vi "InitEqui.vi"(8 "errin":errorcluster, 10 "VISA HITECH":string, 11 "VISA Auto":string) -> (0 "errout":errorcluster, 2 "VisaHitech":refnum<visa-resource-name>, 3 "VISA Refnum out":refnum<visa-resource-name>)   [LabVIEW 2020]
uses:
  <vilib>/Instr/_visa.llb/VISA Configure Serial Port (Instr).vi
  <instrlib>/IT6000C/IT6000C.lvlib
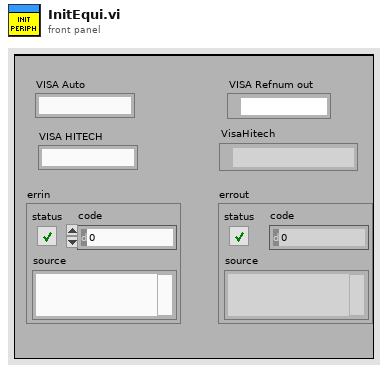
[diagram p1: front panel]
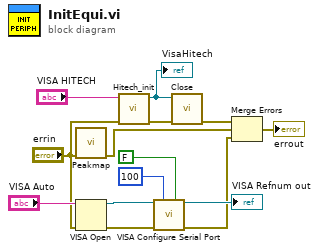
[diagram p0: block diagram]
diagram:
  n1 = call "Peakmap.vi"("errin"="errin") -> ("error out"=w6:errorcluster)  [unwired: 9 in, 1 out]
  n2 = VISA Open(error in (no error)="errin", VISA resource name="VISA Auto") -> (VISA resource name=w11:refnum<visa-resource-name>, error out=w12:errorcluster)  [unwired: 3 in]
  n3 = call "Hitech_init.vi"("errin"="errin", "VISA HITECH"="VISA HITECH") -> ("error out"=w3:errorcluster, "VisaHitech"=w2:refnum<visa-resource-name>)  [unwired: 8 in]
  "VisaHitech" <- w2
  n4 = call-poly "VISA Configure Serial Port"("VISA resource name"=w11, "timeout (10sec)"=u32 100, "Enable Termination\nChar (T)"=FALSE ("Enable Termination\nChar (T)"), "error in (no error)"=w12) -> ("VISA resource name out"=→"VISA Refnum out":refnum<visa-resource-name>, "error out"=w7:errorcluster)  [unwired: 10 in]
  n5 = call <instrlib>:"Close.vi"("error in (no error)"=w3, "VISA resource name"=w2) -> ("error out"=w1:errorcluster)  [unwired: 9 in]
  n6 = Merge Errors(w1, w6, w7) -> (→"errout":errorcluster)
